vi "getUserEvents.vi"(11 "Telemetry in":refnum<class "Telemetry.lvclass">) -> (2 "UserEvents":refnum<class "UserEvents.lvclass">, 3 "Telemetry out":refnum<class "Telemetry.lvclass">)   [LabVIEW 2016, in "Telemetry.lvclass"]
uses:
  Telemetry.lvclass
  UserEvents/UserEvents.lvclass
  Telemetry.lvclass/Telemetry.ctl
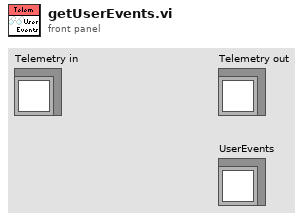
[diagram p1: front panel]
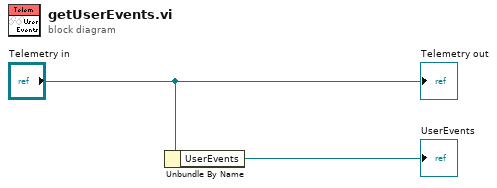
[diagram p0: block diagram]
diagram:
  n1 = Unbundle By Name("Telemetry in") -> ("UserEvents"=→"UserEvents":refnum<class "UserEvents.lvclass">)
  "Telemetry out" <- "Telemetry in"
